vi "dB to volts.vi"(9 "Full scale range":dbl, 11 "Voltage(dB)":dbl) -> (3 "Voltage(volts)":dbl)   [LabVIEW 2021]
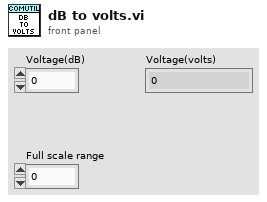
[diagram p1: front panel]
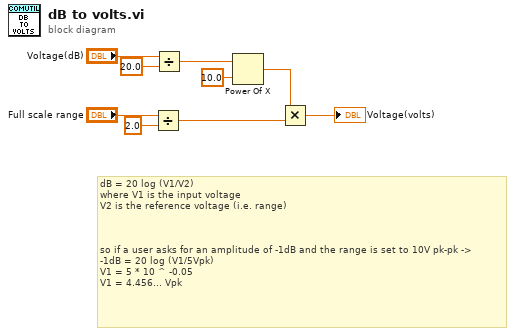
[diagram p0: block diagram]
diagram:
  # "dB = 20 log (V1/V2)\nwhere V1 is the input voltage\nV2 is the reference voltage (i.e. range)\n\n\n\nso if a user asks for an amplitude of -1dB and the range is set to 10V pk-pk ->\n-1dB = 20 log (V1/5Vpk)\nV1 = 5 * 10 ^ -0.05\nV1 = 4.456... Vpk"
  n1 = Divide(x="Full scale range", y=2.0) -> (x/y=w2:dbl)
  n2 = Divide(x="Voltage(dB)", y=20.0) -> (x/y=w4:dbl)
  n3 = Power Of X(1:10.0 ("x"), 2:w4) -> (0:w3:dbl)
  n4 = Multiply(x=w3, y=w2) -> (x*y=→"Voltage(volts)":dbl)
